vi "robotChoosePosition.vi"(10 "RobotRef in":refnum<class "Robot.lvclass">[](array[class]), 11 "sorted 2D array":dbl[][](array[numeric])) -> (3 "Array":refnum<class "Robot.lvclass">[](array[class]))   [LabVIEW 2020, in "Ally.lvclass"]
uses:
  Ally.lvclass
  Robot_class/Robot.lvclass
  f309d3e0-aec7-4123-b46f-518fe36555e2.vi
  <vilib>/Array/Sort 2D Array - Pop Stack.vi
  <vilib>/Array/Sort 2D Array - Push Stack.vi
  f309d3e0-aec7-4123-b46f-518fe36555e2.vi/269d4b3b-47f5-49e3-8884-44851e4dd9d5.vi
  f309d3e0-aec7-4123-b46f-518fe36555e2.vi/6d99389c-673d-4efb-bf33-19b32bcf4cf8.vi
  Ally.lvclass/Ally.ctl
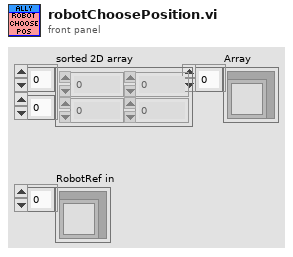
[diagram p1: front panel]
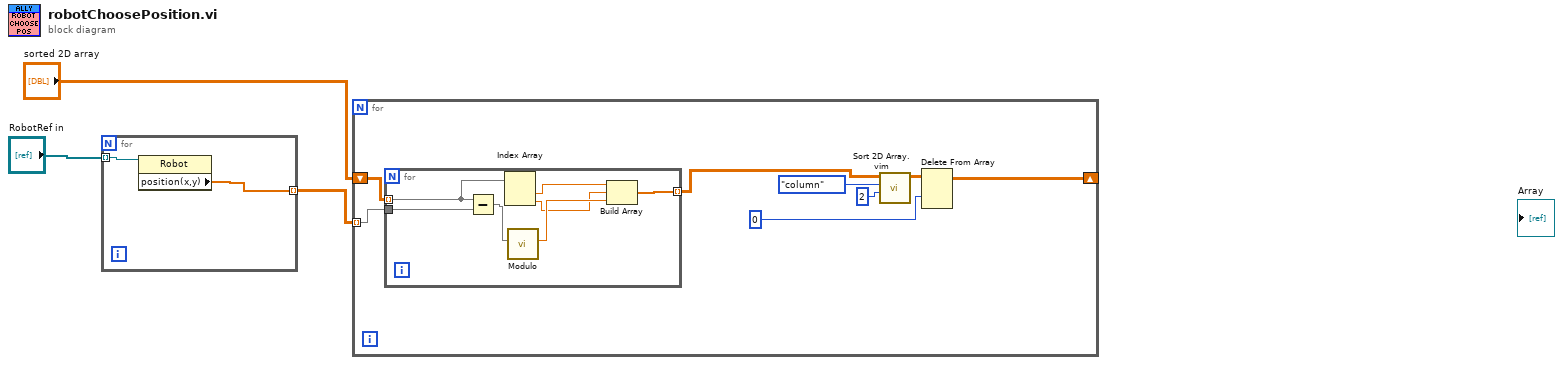
[diagram p0: block diagram]
diagram:
  n1 = for {
    tunnel: "RobotRef in" -> [w5] mode=indexing
    tunnel: [w4] -> w1 mode=indexing
    n2 = property class="Robot"(reference=w5) -> ("position(x,y)"=w4:dbl[])  [unwired: 1 in, 2 out]
  }
  n3 = for {
    shift-right: [w7] -> _
    shift-left: "sorted 2D array" -> [w13]
    tunnel: w1 -> [w6] mode=indexing
    n4 = for {
      tunnel: [w18] -> w9 mode=indexing
      tunnel: w13 -> [w16] mode=indexing
      tunnel: w6 -> [w17]
      n5 = Subtract(x=w16, y=w17) -> (x-y=w19:dbl[])
      n6 = Index Array(array=w16) -> (element #1=w15:dbl, element #2=w14:dbl)  [unwired: 2 in]
      n7 = call "Modulo.vi"("2D vector"=w19) -> ("Modulo"=w20:dbl)  [unwired: 10 in]
      n8 = Build Array(w15, w14, w20) -> (w18:dbl[])
    }
    n9 = call "Sort 2D Array.vim"("index"=2, "dimension to index (column)"=enum16{"column", "row"}."column", "2D array"=w9) -> ("sorted 2D array"=w12:dbl[][])  [unwired: 7 in, 1 out]
    n10 = Delete From Array(array=w12, index (row)=0) -> (array with subset deleted=w7:dbl[][])  [unwired: 2 in, 1 out]
  }
